vi "MainFPGA.vi"() -> ()   [LabVIEW 2019]
uses:
  TypeDefs/TimeSymbol.ctl
  <vilib>/Platform/TimedLoop/XDataNode/timing_clust.ctl
  <vilib>/Platform/TimedLoop/XDataNode/nitl_modes.ctl
  <vilib>/Platform/TimedLoop/XDataNode/wakeup.ctl
  <vilib>/rvi/Emulation/niFpgaGetClockAttributes.vi
  <vilib>/rvi/Emulation/niFpgaSctlEmulationGetInTimedLoop.vi
  <vilib>/rvi/Emulation/niFpgaEmulationReportErrorSimple.vi
  <vilib>/rvi/eio/common/nirviEmuTemplateMethod_errors.vi
  <vilib>/rvi/Emulation/niFpgaCriticalErrorInLSC.vi
  <instrlib>/_niInstr/Basic Elements/v1/FPGA/Private/D Latch U64.vi
  <instrlib>/_niInstr/Basic Elements/v1/FPGA/Private/D Latch U16.vi
  <instrlib>/_niInstr/Basic Elements/v1/FPGA/Private/D Latch U32.vi
  <vilib>/eio/EIONode/EIONode.xnode
  <vilib>/platform/TimedLoop/XDataNode/XDataNode.xnode
  <instrlib>/_niInstr/Basic Elements/v1/FPGA/niInstr Basic Elements v1 FPGA.lvlib
  <vilib>/Platform/TimedLoop/XDataNode/XDNodeRunTimeDep.lvlib
panel:
  in  "Min Pulse":u32 format="%.3p"
  in  "Reset":bool
  out "WWVB":u64 format="%.0x"
  in  "bypasscntr":bool
  in  "Divider":u32=400000 format="%.3p"
  in  "Max Total":u32=50000000 format="%.3p"
  out "OnTime":u32 format="%.3p"
  out "OffTime":u32 format="%.3p"
  out "TotalTime":u32 format="%.3p"
  out "Valid":bool
  out "Symbol":T1=enum."Marker"
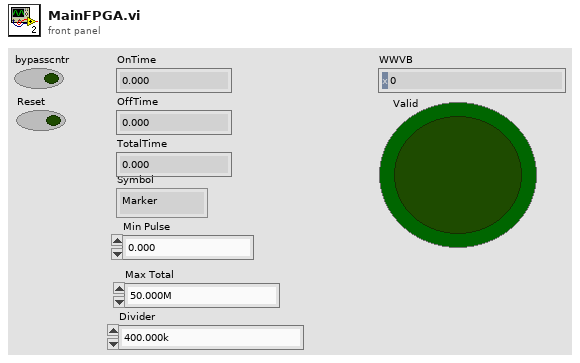
[diagram p1: front panel]
types:
  T1 = typedef "TimeSymbol.ctl" = enum16{"0", "1", "Marker", "Invalid"}
  T2 = typedef "XDNodeRunTimeDep.lvlib/timing_clust.ctl" = cluster{"Expected End [f-1]":u64, "Actual End [f-1]":u64, "Finished Late? [f-1]":bool, "Expected End [i-1]":u64, "Actual End [i-1]":u64, "Finished Late? [i-1]":bool, "Expected Start [i]":u64, "Actual Start [i]":u64, "Expected Start [f]":u64, "Actual Start [f]":u64, "Source Name":string, "Structure Name":string, "Period":i64, "Deadline":i64, "Offset":i64, "Start":i64, "Priority":i32, "Timeout":i32, "Mode":T3, "Wakeup Reason":T4, "Error":errorcluster, "Source Type":string, "Secondary Source Type":string, "Global End Time":u64, "Global Start Time":u64, "Frame Duration":u64, "Iteration Duration":u64, "Assigned CPU":i32, "I/O Scan Engine Mode":u32}
  T3 = typedef "XDNodeRunTimeDep.lvlib/nitl_modes.ctl" = enum32{"No Change", "Process missed periods, maintain original phase", "Discard missed periods, maintain original phase", "Process missed periods, ignore original phase", "Discard missed periods, ignore original phase"}
  T4 = typedef "XDNodeRunTimeDep.lvlib/wakeup.ctl" = enum32{"Normal", "Aborted", "Asynchronous wakeup", "Timing source error", "Timed loop error", "Timeout"}
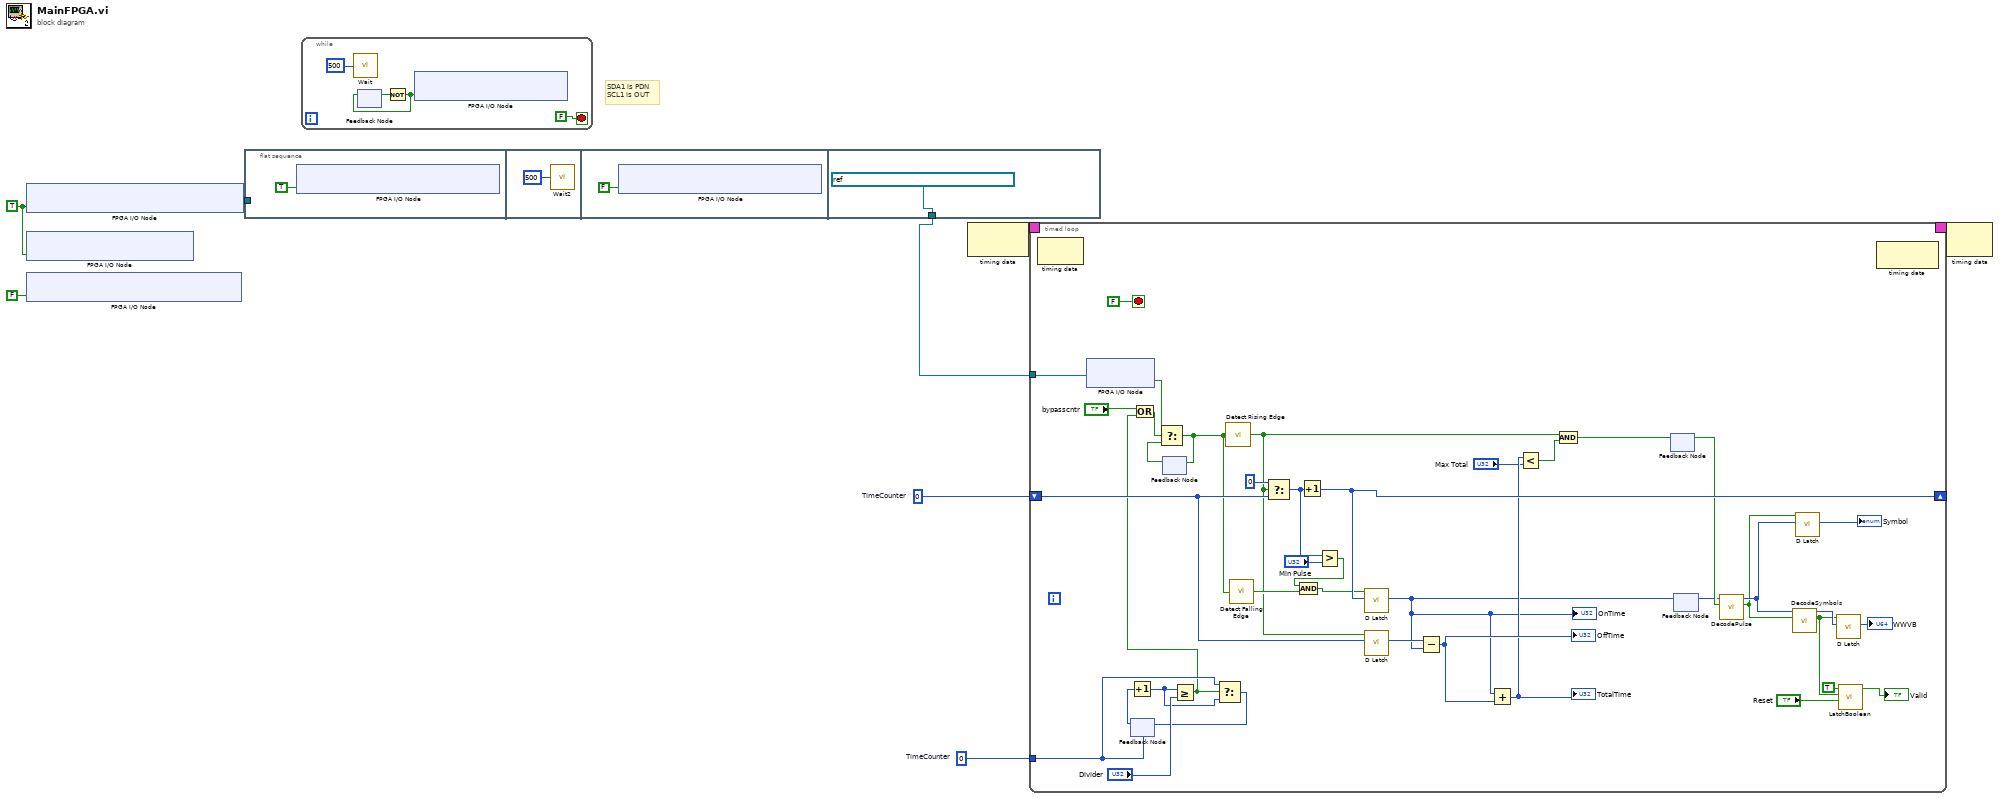
[diagram p0: block diagram]
diagram:
  w1 = u32 0  # TimeCounter
  w3 = u32 0  # TimeCounter
  w8 = TRUE ("sbRIO-9651 Socket\\PMOD_I2C_SDA1_enable")
  # "SDA1 is PDN\nSCL1 is OUT"
  n1 = xnode "FPGA I/O Node"("sbRIO-9651 Socket\\PMOD_I2C_SDA1_enable"=w8) -> ("FPGA I/O Out"=w6:refnum<k21>)  [unwired: 1 in]
  n2 = xnode "FPGA I/O Node"("sbRIO-9651 Socket\\LED1_enable"=w8) -> ()  [unwired: 1 in, 1 out]
  n3 = xnode "FPGA I/O Node"("sbRIO-9651 Socket\\PMOD_I2C_SCL1_enable"=FALSE ("sbRIO-9651 Socket\\PMOD_I2C_SCL1_enable")) -> ()  [unwired: 1 in, 1 out]
  n4 = flat-sequence {
    tunnel: w6 -> [_]
    tunnel: [refnum<k21> "sbRIO-9651 Socket\\PMOD_I2C_SCL1_in" ("FPGA I/O In")] -> w2
    frame #0 {
      n5 = xnode "FPGA I/O Node"("sbRIO-9651 Socket\\PMOD_I2C_SDA1_out"=TRUE ("sbRIO-9651 Socket\\PMOD_I2C_SDA1_out")) -> ()  [unwired: 1 in, 1 out]
    }
    frame #1 {
      n6 = call "Wait2"("Count(mSec)"=u32 500) -> ()  [unwired: 1 out]
    }
    frame #2 {
      n7 = xnode "FPGA I/O Node"("sbRIO-9651 Socket\\PMOD_I2C_SDA1_out"=FALSE ("sbRIO-9651 Socket\\PMOD_I2C_SDA1_out")) -> ()  [unwired: 1 in, 1 out]
    }
    frame #3 {
    }
  }
  n8 = while {
    stop <- FALSE stop-if-true
    n9 = call "Wait"("Count(mSec)"=u32 500) -> ()  [unwired: 1 out]
    n10 = feedback #1() -> (w15:bool)  [unwired: 1 in]
    n11 = Not(x=w15) -> (.not. x?=w14:bool)
    n12 = feedback-in #1(w14) -> ()
    n13 = xnode "FPGA I/O Node"("sbRIO-9651 Socket\\LED1_out"=w14) -> ()  [unwired: 1 in, 1 out]
  }
  n14 = node-c288() -> (w5:T2)  [unwired: 1 in]
  n15 = timed-loop {
    tunnel: w2 -> [w56]
    shift-right: [w54] -> _
    shift-left: w3 -> [w52]
    timing: w5 -> [_]
    timing-out: [_] -> w4
    tunnel: w1 -> [w38]
    stop <- FALSE stop-if-true
    n16 = node-c288() -> ()  [unwired: 1 in, 1 out]
    n17 = xnode "FPGA I/O Node"("FPGA I/O In"=w56) -> ("I/O Item"=w32:bool)  [unwired: 1 out]
    n18 = feedback #2(w38) -> (w40:u32)
    n19 = Increment(x=w40) -> (x+1=w36:u32)
    n20 = feedback #3() -> (w33:bool)  [unwired: 1 in]
    n21 = Greater Or Equal?(x=w36, y="Divider") -> (x >= y?=w35:bool)
    n22 = Or(x="bypasscntr", y=w35) -> (x .or. y?=w31:bool)
    n23 = Select(t=w32, s=w31, f=w33) -> (s? t:f=w34:bool)
    n24 = feedback-in #3(w34) -> ()
    n25 = Select(t=w38, s=w35, f=w36) -> (s? t:f=w37:u32)
    n26 = feedback-in #2(w37) -> ()
    n27 = call <instrlib>:"Detect Rising Edge.vi"("signal"=w34) -> ("edge detected"=w42:bool)  [unwired: 14 in]
    n28 = call <instrlib>:"Detect Falling Edge.vi"("signal"=w34) -> ("edge detected"=w51:bool)  [unwired: 14 in]
    n29 = Select(t=u32 0, s=w42, f=w52) -> (s? t:f=w20:u32)
    n30 = Increment(x=w20) -> (x+1=w54:u32)
    n31 = Greater?(x=w20, y="Min Pulse") -> (0:w17:bool)
    n32 = And(x=w17, y=w51) -> (x .and. y?=w18:bool)
    n33 = call-poly <instrlib>:"D Latch.vi"("d"=w54, "s"=w18) -> ("q"=w45:u32)  [unwired: 9 in]
    "OnTime" <- w45
    n34 = call-poly <instrlib>:"D Latch.vi"("d"=w52, "s"=w42) -> ("q"=w50:u32)  [unwired: 9 in]
    n35 = Subtract(x=w50, y=w45) -> (x-y=w49:u32)
    "OffTime" <- w49
    n36 = Add(x=w45, y=w49) -> (x+y=w48:u32)
    "TotalTime" <- w48
    n37 = Less?(x=w48, y="Max Total") -> (x < y?=w46:bool)
    n38 = And(x=w42, y=w46) -> (x .and. y?=w41:bool)
    n39 = feedback-in #4(w41) -> ()
    n40 = feedback #4() -> (w44:bool)  [unwired: 1 in]
    n41 = feedback-in #5(w45) -> ()
    n42 = feedback #5() -> (w43:u32)  [unwired: 1 in]
    n43 = call "DecodePulse.vi"("ValidInput"=w44, "OnTime"=w43) -> ("OutputValid"=w27:bool, "s? t:f"=w28:T1)  [unwired: 8 in]
    n44 = call "DecodeSymbols.vi"("InputValid"=w27, "Symbol"=w28) -> ("Output Valid"=w24:bool, "WWVB"=w26:u64)  [unwired: 8 in]
    n45 = call-poly <instrlib>:"D Latch.vi"("d"=w28, "s"=w27) -> ("q"=→"Symbol":u16)  [unwired: 9 in]
    n46 = call-poly <instrlib>:"D Latch.vi"("d"=w26, "s"=w24) -> ("q"=→"WWVB":u64)  [unwired: 9 in]
    n47 = call "LatchBoolean.vi"("Reset"="Reset", "Set"=w24, "D"=TRUE) -> ("Q"=→"Valid":bool)  [unwired: 8 in]
    n48 = node-c288() -> ()  [unwired: 1 in, 1 out]
  }
  n49 = node-c288(w4) -> ()  [unwired: 1 out]
